vi "LEP_RV_ReadLine.vi"(2 "error in":errorcluster, 3 "Refnum of LabVIEW.map file":refnum<file>) -> (0 "error out":errorcluster, 1 "Line":string)   [LabVIEW 2011]
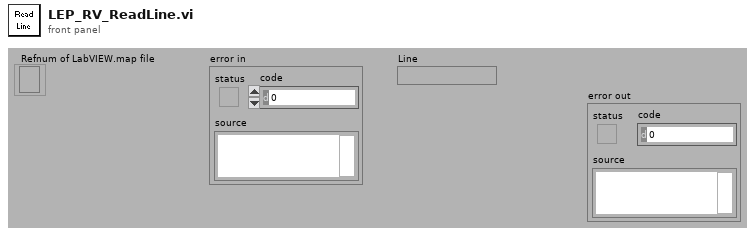
[diagram p1: front panel]
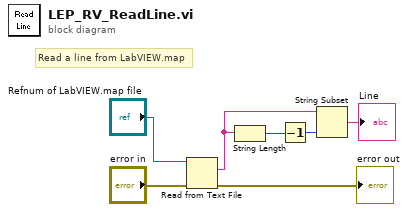
[diagram p0: block diagram]
diagram:
  # "Read a line from LabVIEW.map"
  n1 = Read from Text File(file (use dialog)="Refnum of LabVIEW.map file", error in="error in") -> (text=w5:string, error out=→"error out":errorcluster)  [unwired: 2 in, 2 out]
  n2 = String Length(string=w5) -> (length=w7:i32)
  n3 = Decrement(x=w7) -> (x-1=w6:i32)
  n4 = String Subset(string=w5, length (rest)=w6) -> (substring=→"Line":string)  [unwired: 1 in]
